vi "S2C_VLFT10_Proc_FpButtons.vi"(8 "Error In":errorcluster, 11 "Button":string) -> (0 "Error Out":errorcluster, 3 "Result":string)   [LabVIEW 2015]
uses:
  Controls/VolumeBtn.ctl
  Controls/ServiceBtn.ctl
  Controls/RecallBtn.ctl
  Fornax/VIs/PolyDriver/Typedefs/FrontPanelButtonId.ctl
  Fornax/VIs/PolyDriver/Typedefs/SwitchState.ctl
  Controls/PowerBtn.ctl
  Fornax/VIs/S2C_FORNAX_Proc_Globals.vi
panel:
  in  "Fail":bool
  out "Tab":enum32{"Recall", "Service", "Volume"}(tab)
  out "Recall2":T1
  out "Recall":T1
  out "Service2":T2
  out "Service":T2
  out "Volume2":T3
  out "Volume":T3
  # "Press and Release the shown\nfront panel button \"Twice\""
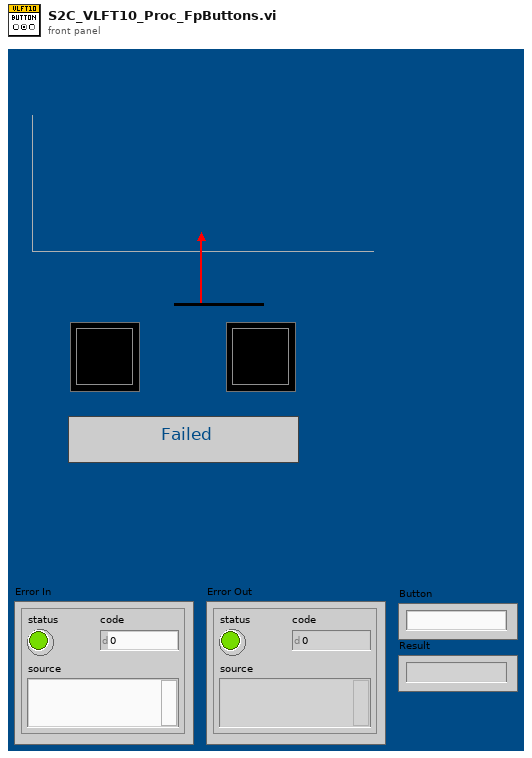
[diagram p1: front panel]
types:
  T1 = typedef "RecallBtn.ctl" = bool
  T2 = typedef "ServiceBtn.ctl" = bool
  T3 = typedef "VolumeBtn.ctl" = bool
  T4 = typedef "FrontPanelButtonId.ctl" = i16
  T5 = typedef "PowerBtn.ctl" = bool
  T6 = typedef "SwitchState.ctl" = i16
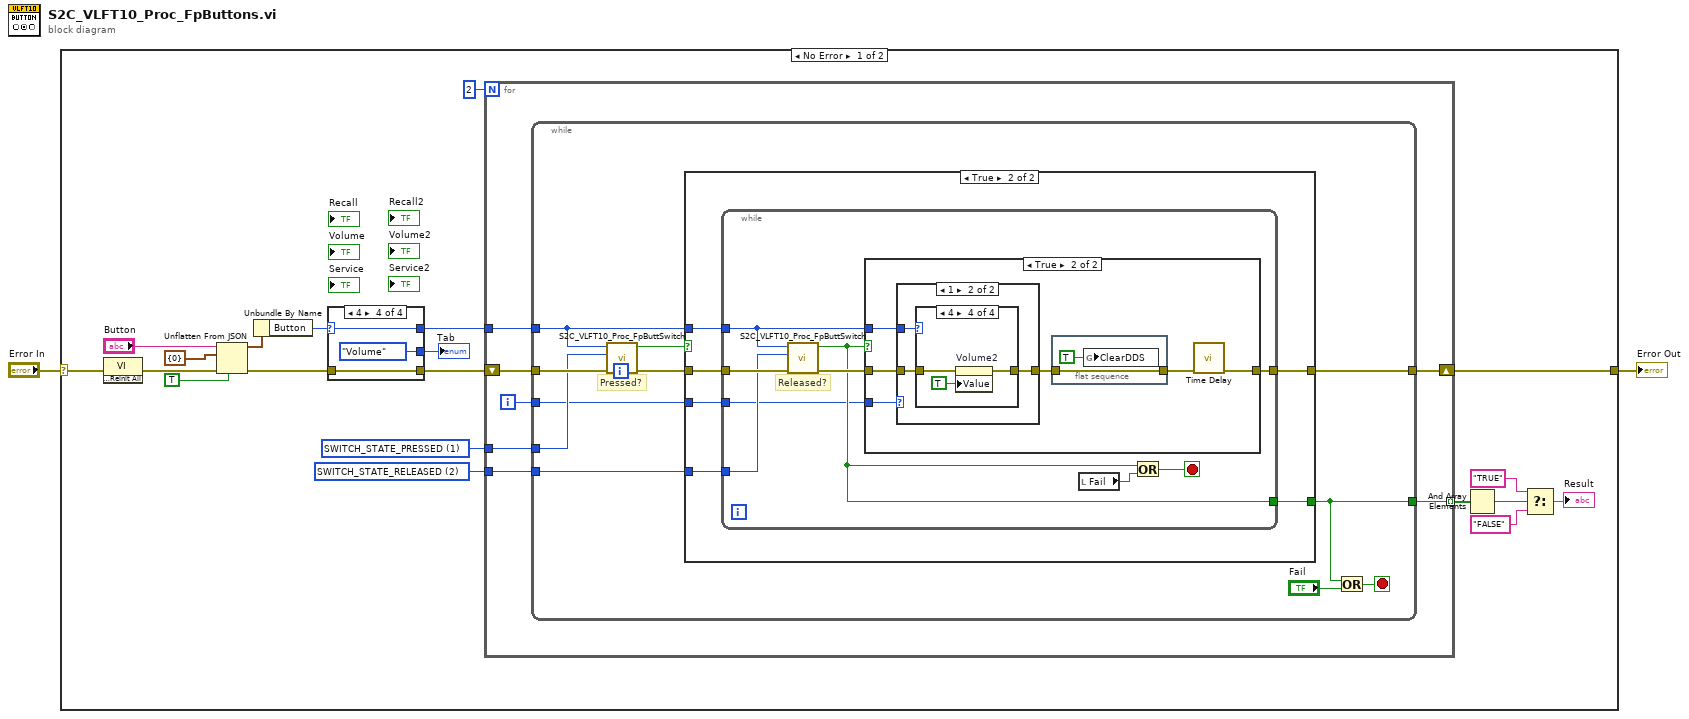
[diagram p0: block diagram]
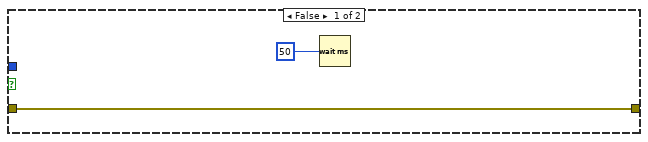
[diagram p2: hidden frame]
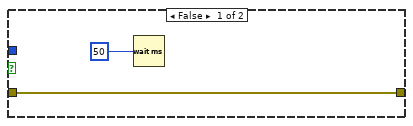
[diagram p3: hidden frame]
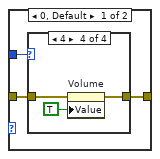
[diagram p4: hidden frame]
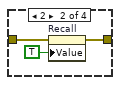
[diagram p6: hidden frame]
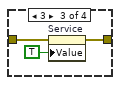
[diagram p7: hidden frame]
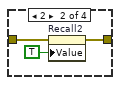
[diagram p9: hidden frame]
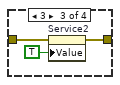
[diagram p10: hidden frame]
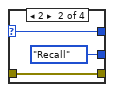
[diagram p12: hidden frame]
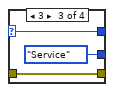
[diagram p13: hidden frame]
diagram:
  n1 = case shown="No Error" "Error In" {
    selector: "Error In" -> [w3 w105]
    tunnel: [w17 w105] -> w2
    frame No Error {
      w18 = T6 2 items=["SWITCH_STATE_NULL", "SWITCH_STATE_PRESSED", "SWITCH_STATE_RELEASED", "NUM_SWITCH_STATES"] ("State")
      w19 = T6 1 items=["SWITCH_STATE_NULL", "SWITCH_STATE_PRESSED", "SWITCH_STATE_RELEASED", "NUM_SWITCH_STATES"] ("State")
      n2 = invoke class="VI" method="Default Vals.Reinit All"(error in=w3) -> (error out=w12:errorcluster)  [unwired: 2 in, 2 out]
      n3 = Unflatten From JSON(JSON string="Button", type and defaults=cluster{"Button":T4} {"Button"=0}, default null elements? (F)=TRUE, error in (no error)=w12) -> (value=w20:cluster{"Button":T4}, error out=w16:errorcluster)  [unwired: 3 in]
      n4 = Unbundle By Name(w20) -> ("Button"=w14:T4)
      n5 = case shown="4" w14 {
        selector: w14 -> [w94 w97 w100 w103]
        tunnel: w16 -> [w95 w98 w101 w104]
        tunnel: [w95 w98 w101 w104] -> w15
        tunnel: [w94 w97 w100 w103] -> w13
        tunnel: [_ enum32{"Recall", "Service", "Volume"}."Recall" ("Tab") enum32{"Recall", "Service", "Volume"}."Service" ("Tab") enum32{"Recall", "Service", "Volume"}."Volume" ("Tab")] -> w10
        frame 0, Default {
        }
        frame 2 {
        }
        frame 3 {
        }
        frame 4 {
        }
      }
      "Tab" <- w10
      n6 = for {
        N: 2 -> [_]
        tunnel: w19 -> [w29]
        tunnel: w18 -> [w28]
        tunnel: w13 -> [w25]
        shift-right: [w27] -> w17
        shift-left: w15 -> [w26]
        tunnel: [w23] -> w9 mode=indexing
        i -> [w24]
        n7 = while {
          tunnel: w26 -> [w40]
          tunnel: w25 -> [w36]
          tunnel: [w34] -> w27
          tunnel: w29 -> [w39]
          tunnel: w28 -> [w35]
          tunnel: w24 -> [w31]
          tunnel: [w30] -> w23
          stop <- w32 stop-if-true
          # "Pressed?"
          n8 = call "S2C_VLFT10_Proc_FpButtSwitch.vi"("Error In"=w40, "State"=w39, "Button"=w36) -> ("Error Out"=w38:errorcluster, "Pass?"=w37:bool)  [unwired: 7 in]
          n9 = case shown="True" w37 {
            tunnel: w38 -> [w41 w48]
            tunnel: w36 -> [_ w47]
            tunnel: w35 -> [_ w46]
            tunnel: [w41 w45] -> w34
            tunnel: [_ w44] -> w30
            tunnel: w31 -> [_ w43]
            frame False {
              n10 = Wait (ms)(milliseconds to wait=u32 50) -> ()  [unwired: 1 out]
            }
            frame True {
              n11 = while {
                tunnel: w48 -> [w57]
                tunnel: w47 -> [w54]
                tunnel: w46 -> [w56]
                tunnel: [w53] -> w45
                tunnel: [w51] -> w44
                tunnel: w43 -> [w49]
                stop <- w52 stop-if-true
                # "Released?"
                n12 = call "S2C_VLFT10_Proc_FpButtSwitch.vi"("Error In"=w57, "State"=w56, "Button"=w54) -> ("Error Out"=w55:errorcluster, "Pass?"=w51:bool)  [unwired: 7 in]
                n13 = case shown="True" w51 {
                  tunnel: w55 -> [w59 w65]
                  tunnel: w54 -> [_ w64]
                  tunnel: [w59 w61] -> w53
                  tunnel: w49 -> [_ w60]
                  frame False {
                    n14 = Wait (ms)(milliseconds to wait=u32 50) -> ()  [unwired: 1 out]
                  }
                  frame True {
                    n15 = case shown="1" w60 {
                      tunnel: w65 -> [w68 w81]
                      tunnel: w64 -> [w67 w80]
                      tunnel: [w66 w79] -> w63
                      frame 0, Default {
                        n16 = case shown="4" w67 {
                          tunnel: w68 -> [w69 w72 w75 w78]
                          tunnel: [w69 w71 w74 w77] -> w66
                          frame 0, Default {
                          }
                          frame 2 {
                            n17 = property on="Recall" class="Bool (strict)"(error in=w72, "Value"=T5 TRUE ("Power1")) -> (error out=w71:errorcluster)  [unwired: 1 in, 1 out]
                          }
                          frame 3 {
                            n18 = property on="Service" class="Bool (strict)"(error in=w75, "Value"=T5 TRUE ("Power1")) -> (error out=w74:errorcluster)  [unwired: 1 in, 1 out]
                          }
                          frame 4 {
                            n19 = property on="Volume" class="Bool (strict)"(error in=w78, "Value"=T5 TRUE ("Power1")) -> (error out=w77:errorcluster)  [unwired: 1 in, 1 out]
                          }
                        }
                      }
                      frame 1 {
                        n20 = case shown="4" w80 {
                          tunnel: w81 -> [w82 w85 w88 w91]
                          tunnel: [w82 w84 w87 w90] -> w79
                          frame 0, Default {
                          }
                          frame 2 {
                            n21 = property on="Recall2" class="Bool (strict)"(error in=w85, "Value"=T5 TRUE ("Power1")) -> (error out=w84:errorcluster)  [unwired: 1 in, 1 out]
                          }
                          frame 3 {
                            n22 = property on="Service2" class="Bool (strict)"(error in=w88, "Value"=T5 TRUE ("Power1")) -> (error out=w87:errorcluster)  [unwired: 1 in, 1 out]
                          }
                          frame 4 {
                            n23 = property on="Volume2" class="Bool (strict)"(error in=w91, "Value"=T5 TRUE ("Power1")) -> (error out=w90:errorcluster)  [unwired: 1 in, 1 out]
                          }
                        }
                      }
                    }
                    n24 = flat-sequence {
                      tunnel: w63 -> [w93]
                      tunnel: [w93] -> w62
                      frame #0 {
                        n25 = global write "S2C_FORNAX_Proc_Globals.vi" "ClearDDS"(TRUE ("ClearDDS")) -> ()
                      }
                    }
                    n26 = call "Time Delay"("error in (no error)"=w62) -> ("error out"=w61:errorcluster)  [unwired: 10 in]
                  }
                }
                n27 = local read "Fail"() -> (w50:bool)
                n28 = Or(x=w51, y=w50) -> (x .or. y?=w52:bool)
              }
            }
          }
          n29 = Or(x=w30, y="Fail") -> (x .or. y?=w32:bool)
        }
      }
      n30 = And Array Elements(Boolean array=w9) -> (logical AND=w7:bool)
      n31 = Select(t="TRUE", s=w7, f="FALSE") -> (s? t:f=→"Result":string)
    }
    frame Error {
    }
  }
  "Error Out" <- w2
